vi "IIC Write Read Bytes.vi"(0 "DevHandle":i32, 1 "WriteLen":i32, 2 "ReadLen":i32, 5 "IICIndex":i32, 7 "SlaveAddr":i16, 9 "pWriteData":u8[](array[numeric])=array[4097 elements], 12 "pReadData":u8[](array[numeric])=array[4097 elements], 13 "TimeOutMs":i32) -> (4 "function return":i32, 10 "pWriteData out":u8[](array[numeric]), 14 "pReadData out":u8[](array[numeric]))   [LabVIEW 2010, in "usb2iic.lvlib"]
doc: "int WINAPI IIC_WriteReadBytes(int DevHandle,int IICIndex,short SlaveAddr,unsigned char *pWriteData,int WriteLen,unsigned char *pReadData,int ReadLen,int TimeOutMs);"
uses:
  usb2iic.lvlib
  USB2XXX.dll
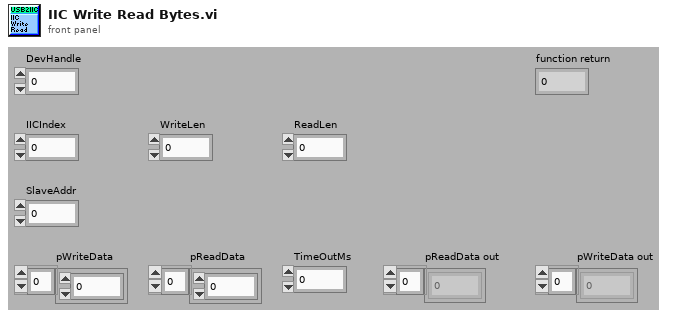
[diagram p1: front panel]
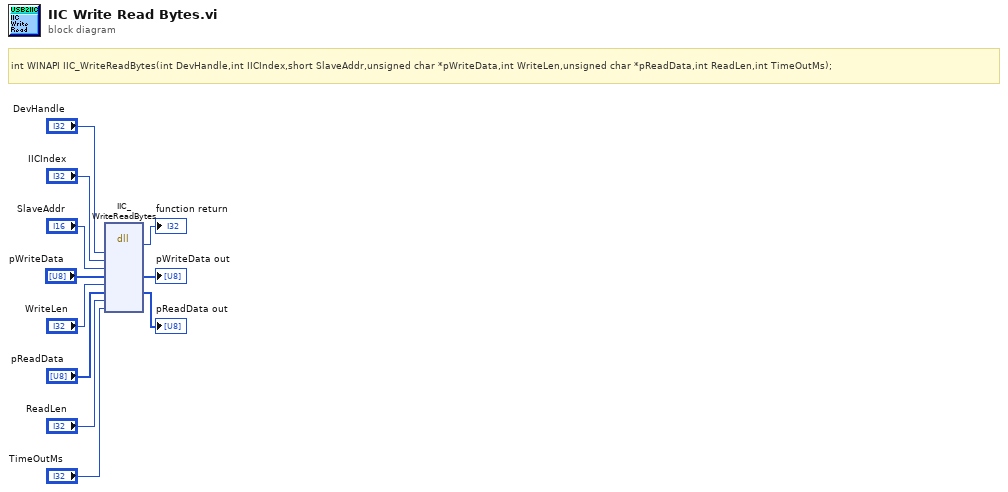
[diagram p0: block diagram]
diagram:
  # "int WINAPI IIC_WriteReadBytes(int DevHandle,int IICIndex,short SlaveAddr,unsigned char *pWriteData,int WriteLen,unsigned char *pReadData,int ReadLen,int TimeOutMs);"
  n1 = dll-call lib="G:/OtherWork/USB2XXX_Example/trunk/Labview/PublicFiles/USB2XXX.*" fn="IIC_WriteReadBytes"("DevHandle"="DevHandle", "IICIndex"="IICIndex", "SlaveAddr"="SlaveAddr", "pWriteData"="pWriteData", "WriteLen"="WriteLen", "pReadData"="pReadData", "ReadLen"="ReadLen", "TimeOutMs"="TimeOutMs") -> (→"function return":i32, "pWriteData"=→"pWriteData out":u8[], "pReadData"=→"pReadData out":u8[])  [unwired: 9 in, 2 out]
